vi "GFITS_GetKeyValue.vi"(8 "error in (no error)":errorcluster, 10 "keyname":string, 11 "action":enum16{"get", "clear"}(ring)) -> (0 "error out":errorcluster, 2 "response":string)   [LabVIEW 2016]
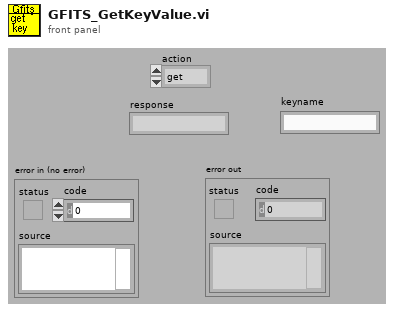
[diagram p1: front panel]
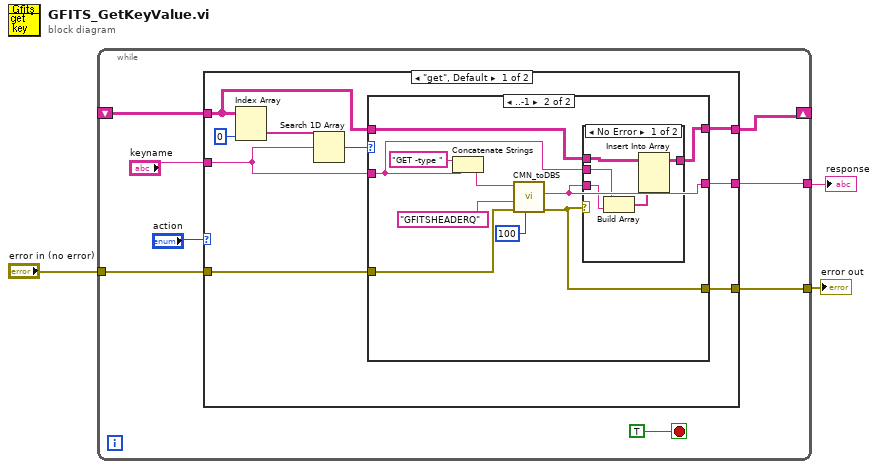
[diagram p0: block diagram]
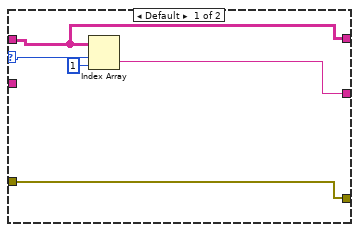
[diagram p2: hidden frame]
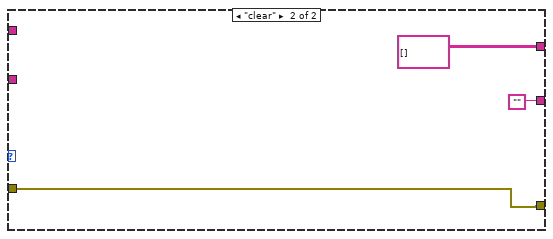
[diagram p4: hidden frame]
diagram:
  n1 = while {
    shift-right: [w7] -> _
    shift-left: _ -> [w9]
    tunnel: "error in (no error)" -> [w6]
    tunnel: [w5] -> w2
    tunnel: [w4] -> w1
    stop <- TRUE stop-if-true
    n2 = case shown="\"get\", Default" "action" {
      tunnel: w9 -> [w14 _]
      tunnel: "keyname" -> [w17 _]
      tunnel: [w12 string[][] [] ("Table")] -> w7
      tunnel: w6 -> [w16 w42]
      tunnel: [w15 w42] -> w5
      tunnel: [w13 ""] -> w4
      frame "get", Default {
        n3 = Index Array(array=w14, index (col)=0 ("disabled index (col)")) -> (element=w19:string[])  [unwired: 1 in]
        n4 = Search 1D Array(1D array=w19, element=w17) -> (index of element=w18:i32)  [unwired: 1 out]
        n5 = case shown="..-1" w18 {
          selector: w18 -> [w25 _]
          tunnel: w14 -> [w24 w29]
          tunnel: w17 -> [_ w27]
          tunnel: w16 -> [w23 w31]
          tunnel: [w23 w30] -> w15
          tunnel: [w21 w28] -> w13
          tunnel: [w24 w26] -> w12
          frame Default {
            n6 = Index Array(array=w24, index (row)=w25, index (col)=1 ("disabled index (col)")) -> (element=w21:string)
          }
          frame ..-1 {
            n7 = Concatenate Strings("GET -type ", w27) -> (w32:string)
            n8 = call "CMN_toDBS.vi"("ms timeout (-1)"=100, "error in (no error)"=w31, "response Q"="GFITSHEADERQ", "command"=w32) -> ("error out"=w30:errorcluster, "response"=w28:string)  [unwired: 6 out]
            n9 = case shown="No Error" w30 {
              tunnel: w29 -> [w40 w41]
              tunnel: w28 -> [w38 _]
              tunnel: w27 -> [w39 _]
              tunnel: [w36 w41] -> w26
              frame No Error {
                n10 = Build Array(w39, w38) -> (w37:string[])
                n11 = Insert Into Array(array=w40, new element=w37) -> (w36:string[][])  [unwired: 2 in]
              }
              frame Error {
              }
            }
          }
        }
      }
      frame "clear" {
      }
    }
  }
  "error out" <- w2
  "response" <- w1
